vi "Pre_Session.vi"(6 "expId":string, 7 "session exists?":bool, 8 "error in (no error)":errorcluster, 9 "expIndex":i32, 10 "Session_timeout":u32, 11 "Web Request in":refnum<class "Web Request.lvclass">) -> (0 "error out":errorcluster, 1 "millisecond timer value":u32, 2 "String":string, 3 "Web Request out":refnum<class "Web Request.lvclass">, 4 "Numeric 2":dbl, 5 "Numeric":u32)   [LabVIEW 2020]
uses:
  <vilib>/wsapi/Web Request.lvclass
  <vilib>/wsapi/class/subVIs/Write Integer Session Variable.vi
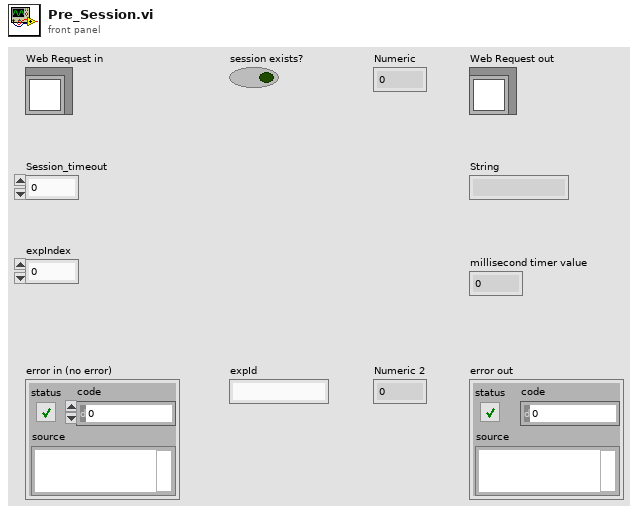
[diagram p1: front panel]
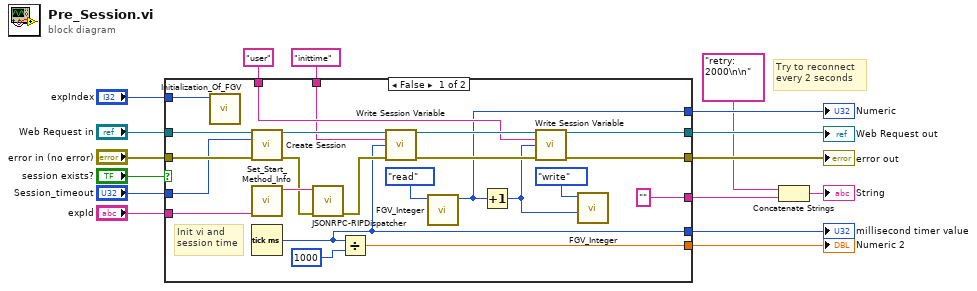
[diagram p0: block diagram]
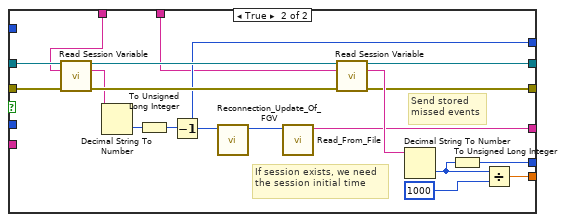
[diagram p2: hidden frame]
diagram:
  # "Try to reconnect \nevery 2 seconds"
  n1 = case shown="False" "session exists?" {
    tunnel: "Web Request in" -> [w39 w48]
    tunnel: [w18 w51] -> w12
    tunnel: "error in (no error)" -> [w38 w46]
    tunnel: [w19 w56] -> w11
    tunnel: "Session_timeout" -> [w37 _]
    tunnel: "expId" -> [w36 _]
    tunnel: [w29 w54] -> w9
    tunnel: [w30 w53] -> w13
    tunnel: ["" ("Events") w42] -> w4
    tunnel: [w20 w43] -> w15
    tunnel: "user" ("key") -> [w23 w41]
    tunnel: "inittime" ("key") -> [w22 w40]
    tunnel: "expIndex" -> [w21 _]
    frame False {
      # "Init vi and \nsession time"
      n2 = call "Initialization_Of_FGV.vi"("expIndex"=w21) -> ()  [unwired: 11 in]
      n3 = call <vilib>:"Create Session.vi"("LabVIEW Web Service Request"=w39, "timeout (60000 msec)"=w37, "error in (no error)"=w38) -> ("LabVIEW Web Service Request out"=w33:refnum<class "Web Request.lvclass">, "error out"=w34:errorcluster)  [unwired: 10 in, 1 out]
      n4 = call "Set_Start_Method_Info.vi"("expId"=w36) -> ("String"=w35:string)  [unwired: 10 in]
      n5 = Tick Count (ms)() -> (millisecond timer value=w30:u32)
      n6 = call "JSONRPC-RIPDispatcher.vi"("error in"=w34, "input string"=w35) -> ("error out"=w32:errorcluster)  [unwired: 8 in, 1 out]
      n7 = Divide(x=w30, y=u32 1000) -> (x/y=w29:dbl)
      n8 = call-poly <vilib>:"Write Session Variable.vi"("LabVIEW Web Service Request"=w33, "key"=w22, "value"=w30, "error in (no error)"=w32) -> ("LabVIEW Web Service Request out"=w27:refnum<class "Web Request.lvclass">, "error out"=w26:errorcluster)  [unwired: 8 in, 2 out]
      n9 = call "FGV_Integer.vi"("Enum"=enum16{"read", "write"}."read") -> ("intout"=w20:i32)  [unwired: 10 in]
      n10 = Increment(x=w20) -> (x+1=w24:i32)
      n11 = call-poly <vilib>:"Write Session Variable.vi"("LabVIEW Web Service Request"=w27, "key"=w23, "value"=w24, "error in (no error)"=w26) -> ("LabVIEW Web Service Request out"=w18:refnum<class "Web Request.lvclass">, "error out"=w19:errorcluster)  [unwired: 8 in, 2 out]
      n12 = call "FGV_Integer.vi"("intin"=w24, "Enum"=enum16{"read", "write"}."write") -> ()  [unwired: 9 in, 1 out]
    }
    frame True {
      # "If session exists, we need the session initial time"
      # "Send stored \nmissed events"
      n13 = call <vilib>:"Read Session Variable.vi"("LabVIEW Web Service Request"=w48, "key"=w41, "error in (no error)"=w46) -> ("LabVIEW Web Service Request out"=w47:refnum<class "Web Request.lvclass">, "value"=w44:string, "error out"=w45:errorcluster)  [unwired: 10 in]
      n14 = Decimal String To Number(string=w44) -> (number=w50:i32)  [unwired: 2 in, 1 out]
      n15 = To Unsigned Long Integer(number=w50) -> (unsigned 32bit integer=w49:u32)
      n16 = Decrement(x=w49) -> (x-1=w43:u32)
      n17 = call "Reconnection_Update_Of_FGV.vi"("user"=w43) -> ()  [unwired: 11 in]
      n18 = call "Read_From_File.vi"("user"=w43) -> ("Events"=w42:string)  [unwired: 9 in, 1 out]
      n19 = call <vilib>:"Read Session Variable.vi"("LabVIEW Web Service Request"=w47, "key"=w40, "error in (no error)"=w45) -> ("LabVIEW Web Service Request out"=w51:refnum<class "Web Request.lvclass">, "value"=w57:string, "error out"=w56:errorcluster)  [unwired: 10 in]
      n20 = Decimal String To Number(string=w57) -> (number=w52:i32)  [unwired: 2 in, 1 out]
      n21 = To Unsigned Long Integer(number=w52) -> (unsigned 32bit integer=w53:u32)
      n22 = Divide(x=w52, y=u32 1000) -> (x/y=w54:dbl)
    }
  }
  "Numeric" <- w15
  "millisecond timer value" <- w13
  "Web Request out" <- w12
  "error out" <- w11
  "Numeric 2" <- w9
  n23 = Concatenate Strings("retry: 2000\n\n" ("response string"), w4) -> (→"String":string)
